vi "solar_qtimer Set Start Target.vi"(6 "Suppress Errors? (T)":bool=TRUE, 8 "error in (no error)":errorcluster, 10 "Target (Queue Name)":string, 11 "QTimer Refnum in":T1) -> (0 "error out":errorcluster, 1 "Previously Running":bool[](array[boolean]), 2 "Target QTimers":string[](array[string]), 3 "QTimer Refnum out":T1)   [LabVIEW 2018]
doc: "This starts all QTimers associated the targets queue name (i.e. Destination queue name = target name). The <b>Target QTimers</b> list the QTimers associated with the target."
uses:
  solar_qtimer_ctl Refnum.ctl
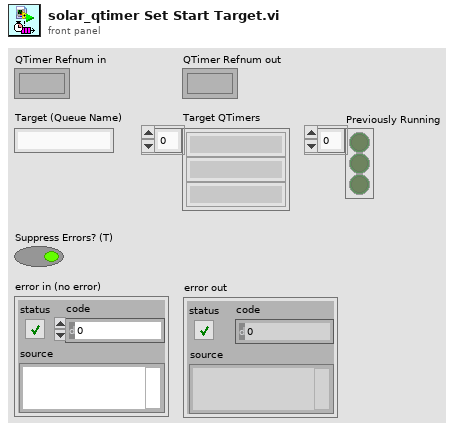
[diagram p1: front panel]
types:
  T1 = typedef "solar_qtimer_ctl Refnum.ctl" = refnum<k1>
  T2 = typedef "solar_qtimer_ctl SEQ.ctl" = cluster{"QTimers":T3[]}
  T3 = typedef "solar_qtimer_ctl QTimer.ctl" = cluster{"Settings":T4, "Queue":refnum<queue>, "QTimerQ":refnum<queue>, "VI Refnum":refnum<vi>}
  T4 = typedef "solar_qtimer_ctl QTimer Settings.ctl" = cluster{"QTimer":string, "Delay":i32, "Start":bool, "EnQ_Type":enum8{"Normal", "Priority", "IgnoreIfExists"}, "Messages":cluster{"MSG":string, "DATA":variant}[]}
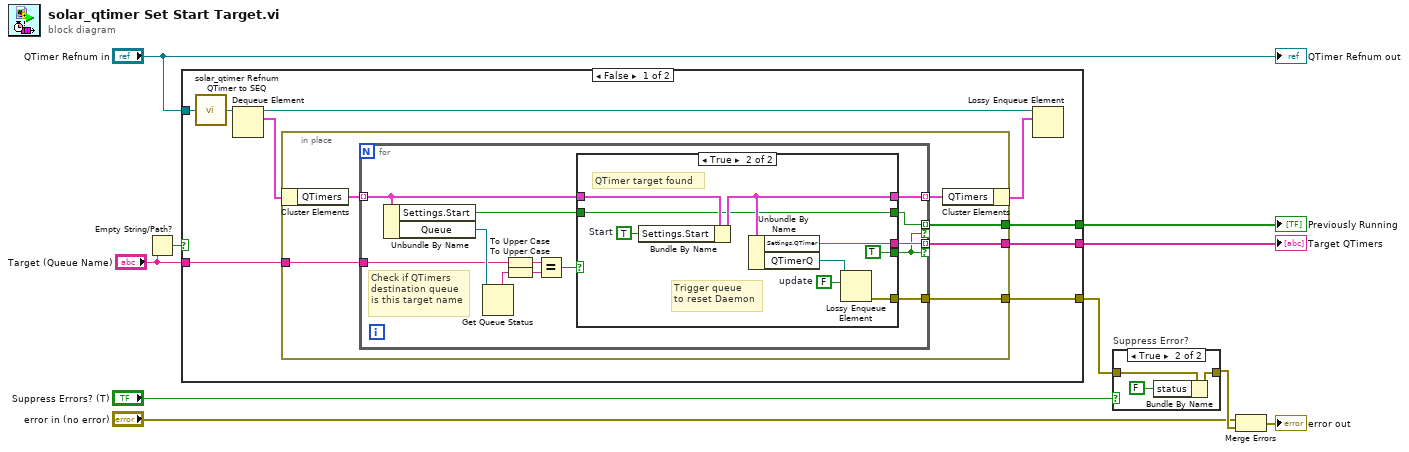
[diagram p0: block diagram]
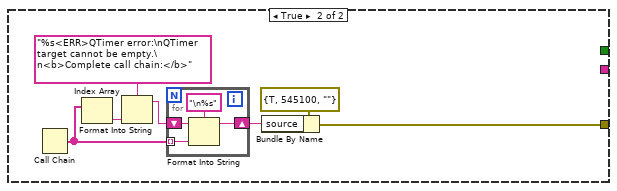
[diagram p3: hidden frame]
diagram:
  n1 = Empty String/Path?(string/path="Target (Queue Name)") -> (empty?=w1:bool)
  n2 = case shown="False" w1 {
    tunnel: "QTimer Refnum in" -> [w19 _]
    tunnel: [w14 w49] -> w7
    tunnel: [w13 _] -> w4
    tunnel: [w12 _] -> w3
    tunnel: "Target (Queue Name)" -> [w11 _]
    frame False {
      n3 = call "solar_qtimer Refnum QTimer to SEQ.vi"("QTimer Refnum"=w19) -> ("QTimers SEQ"=w18:refnum<queue>)
      n4 = Dequeue Element(queue=w18) -> (queue out=w17:refnum<queue>, element=w16:T2)  [unwired: 2 in, 2 out]
      n5 = in-place {
        in-place-border: [w23] -> w14
        in-place-border: [w22] -> w13
        in-place-border: [w21] -> w12
        in-place-border: w11 -> [w20]
        n6 = in-place-cluster #1(w16) -> ("QTimers"=w25:T3[])
        n7 = for {
          tunnel: [w38] -> w23
          tunnel: w25 -> [w35] mode=indexing
          tunnel: [w36] -> w24 mode=indexing
          tunnel: [w37] -> w22 mode=indexing if=w26
          tunnel: [w28] -> w21 mode=indexing if=w26
          tunnel: w20 -> [w33]
          # "Check if QTimers\ndestination queue\nis this target name"
          n8 = Unbundle By Name(w35) -> ("Settings.Start"=w27:bool, "Queue"=w34:refnum<queue>)
          n9 = Get Queue Status(queue=w34) -> (queue name=w32:string)  [unwired: 2 in, 7 out]
          n10 = To Upper Case(1:w33) -> (0:w31:string)
          n11 = To Upper Case(1:w32) -> (0:w30:string)
          n12 = Equal?(x=w31, y=w30) -> (x = y?=w29:bool)
          n13 = case shown="True" w29 {
            tunnel: [_ w42] -> w38
            tunnel: [_ w48] -> w37
            tunnel: [w39 w47] -> w36
            tunnel: w35 -> [w39 w45]
            tunnel: [_ w44] -> w28
            tunnel: w27 -> [_ w44]
            tunnel: [_ TRUE] -> w26
            frame False {
            }
            frame True {
              w46 = TRUE  # Start
              w40 = FALSE  # update
              # "QTimer target found"
              # "Trigger queue\nto reset Daemon"
              n14 = Bundle By Name(cluster=w45, "Settings.Start"=w46) -> (w47:T3)
              n15 = Unbundle By Name(w47) -> ("Settings.QTimer"=w48:string, "QTimerQ"=w41:refnum<queue>)
              n16 = Lossy Enqueue Element(queue=w41, element=w40) -> (error out=w42:errorcluster)  [unwired: 1 in, 3 out]
            }
          }
        }
        n17 = in-place-cluster #1("QTimers"=w24) -> (w15:T2)
      }
      n18 = Lossy Enqueue Element(queue=w17, element=w15) -> ()  [unwired: 1 in, 4 out]
    }
    frame True {
      n19 = Call Chain() -> (call chain=w52:string[])
      n20 = Index Array(array=w52) -> (element=w54:string)  [unwired: 1 in]
      n21 = Format Into String(format string="%s<ERR>QTimer error:\nQTimer target cannot be empty.\n<b>Complete call chain:</b>", w54) -> (resulting string=w53:string)  [unwired: 2 in, 1 out]
      n22 = for {
        tunnel: w52 -> [w59] mode=indexing
        shift-right: [w58] -> w51
        shift-left: w53 -> [w57]
        n23 = Format Into String(format string="\n%s", initial string=w57, w59) -> (resulting string=w58:string)  [unwired: 1 in, 1 out]
      }
      n24 = Bundle By Name(cluster=errorcluster {"status"=TRUE, "code"=545100, "source"=""} ("error in (no error)"), "source"=w51) -> (w49:errorcluster)
    }
  }
  "Target QTimers" <- w4
  "Previously Running" <- w3
  n25 = case "Suppress Error?" shown="True" "Suppress Errors? (T)" {
    tunnel: w7 -> [w60 w63]
    tunnel: [w60 w62] -> w8
    frame False {
    }
    frame True {
      n26 = Bundle By Name(cluster=w63, "status"=FALSE) -> (w62:errorcluster)
    }
  }
  n27 = Merge Errors("error in (no error)", w8) -> (→"error out":errorcluster)
  "QTimer Refnum out" <- "QTimer Refnum in"
